vi "GoBack.vi"(0 "reference in":refnum<class "LcWebView.lvclass">, 5 "Error In":errorcluster) -> (14 "reference out":refnum<class "LcWebView.lvclass">, 19 "Error Out":errorcluster)   [LabVIEW 2018, in "LcWebView.lvclass"]
uses:
  LcWebView.lvclass
  D:/GitProjects/Public/GitHub/LcWebView/data/Microsoft.Web.WebView2.Core.dll
  data/Microsoft.Web.WebView2.Core.dll
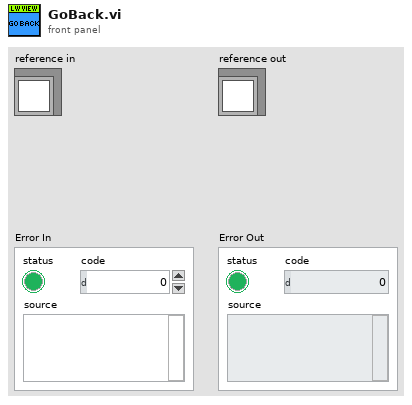
[diagram p1: front panel]
types:
  T1 = typedef "LcWebView.lvclass/ObjectAttributes.ctl" = cluster{"WebView Container":refnum<k24>, "CoreWebViewRef":refnum<k24>, "Status":i32, "Status Message":string, "User Data Folder":path, "BrowserProcessId":u32, "PlotType":T2, "Chart Collection":T3}
  T2 = typedef "LcWebView.lvclass/PlotType.ctl" = enum16{"bar", "line", "pie"}
  T3 = typedef "LcWebView.lvclass/ChartCollection.ctl" = T4[]
  T4 = typedef "LcWebView.lvclass/ChartContent.ctl" = cluster{"Chart Id":string, "Chart Setup":T5, "Chart HTML":string, "Chart Config":string, "Chart Data":string}
  T5 = typedef "LcWebView.lvclass/ChartSetup.ctl" = cluster{"Chart Id":string, "width":u32, "height":u32}
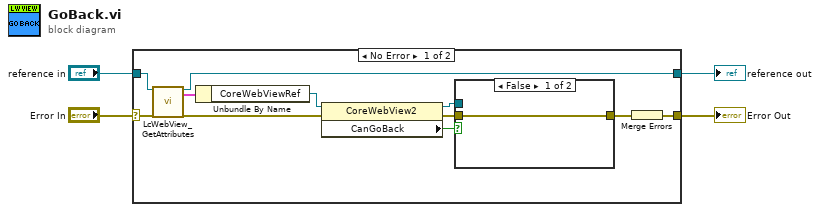
[diagram p0: block diagram]
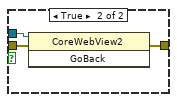
[diagram p2: hidden frame]
diagram:
  n1 = case shown="No Error" "Error In" {
    selector: "Error In" -> [w15 w21]
    tunnel: [w12 w21] -> w3
    tunnel: [w13 w20] -> w1
    tunnel: "reference in" -> [w14 w20]
    frame No Error {
      n2 = call "LcWebView_GetAttributes.vi"("reference in"=w14, "error in (no error)"=w15) -> ("reference out"=w13:refnum<class "LcWebView.lvclass">, "Data"=w11:T1, "error out"=w7:errorcluster)  [unwired: 14 in, 1 out]
      n3 = Unbundle By Name(w11) -> ("CoreWebViewRef"=w9:refnum<k24>)
      n4 = property class="CoreWebView2"(reference=w9, error in=w7) -> (reference out=w8:refnum<k24>, error out=w6:errorcluster, "CanGoBack"=w5:bool)
      n5 = case shown="False" w5 {
        tunnel: [w16 w19] -> w10
        tunnel: w8 -> [_ w18]
        tunnel: w6 -> [w16 w17]
        frame False {
        }
        frame True {
          n6 = invoke class="CoreWebView2" method="GoBack"(reference=w18, error in=w17) -> (error out=w19:errorcluster)  [unwired: 1 in, 2 out]
        }
      }
      n7 = Merge Errors(w10) -> (w12:errorcluster)
    }
    frame Error {
    }
  }
  "Error Out" <- w3
  "reference out" <- w1
